vi "Write Timeout.vi"(8 "error in (no error)":errorcluster, 10 "Timeout":dbl, 11 "Lamp in":refnum<class "Lamp.lvclass">) -> (0 "error out":errorcluster, 3 "Lamp out":refnum<class "Lamp.lvclass">)   [LabVIEW 2016, in "Lamp.lvclass"]
uses:
  Lamp.lvclass
  Lamp.lvclass/Lamp.ctl
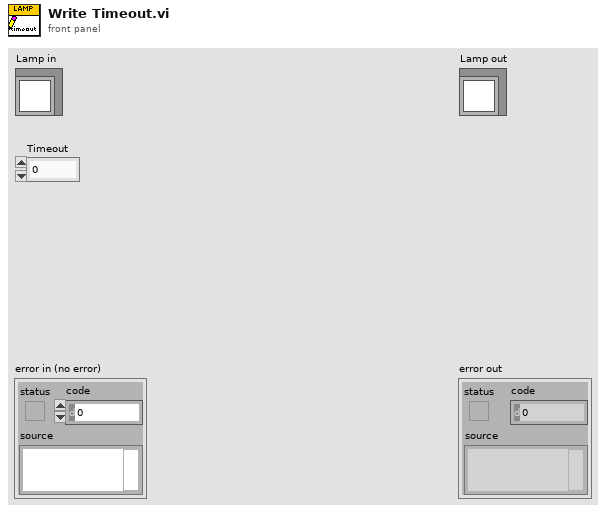
[diagram p1: front panel]
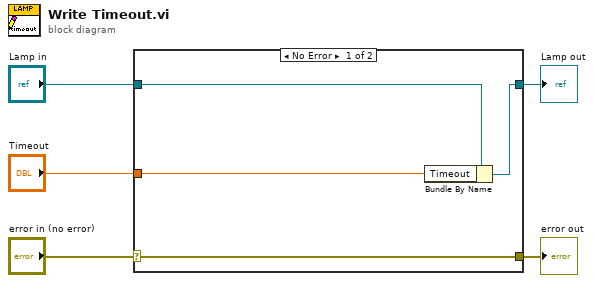
[diagram p0: block diagram]
diagram:
  n1 = case shown="No Error" "error in (no error)" {
    selector: "error in (no error)" -> [w9 w10]
    tunnel: [w9 w10] -> w4
    tunnel: [w7 w11] -> w2
    tunnel: "Lamp in" -> [w8 w11]
    tunnel: "Timeout" -> [w6 _]
    frame No Error {
      n2 = Bundle By Name(cluster=w8, "Timeout"=w6) -> (w7:refnum<class "Lamp.lvclass">)
    }
    frame Error {
    }
  }
  "error out" <- w4
  "Lamp out" <- w2
